vi "Setup subWorker - FPGA Read.vi"(8 "error in":errorcluster, 11 "cRIO NI 9205 Demo in":refnum<class "cRIO NI 9205 Demo.lvclass">) -> (0 "error out":errorcluster, 3 "cRIO NI 9205 Demo out":refnum<class "cRIO NI 9205 Demo.lvclass">)   [LabVIEW 2017, in "cRIO NI 9205 Demo.lvclass"]
doc: "This VI sets up the framework parameters of a statically-linked subWorker."
uses:
  cRIO NI 9205 Demo.lvclass
  cRIO NI 9205 Demo.lvclass/cRIO NI 9205 Demo.ctl
  FPGA Read/FPGA Read.lvclass
  C:/Program Files (x86)/National Instruments/LabVIEW 2017/vi.lib/addons/_Workers/Library/Classes/Worker/Worker.lvclass
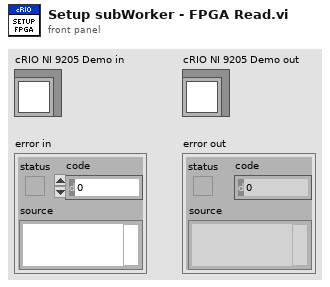
[diagram p1: front panel]
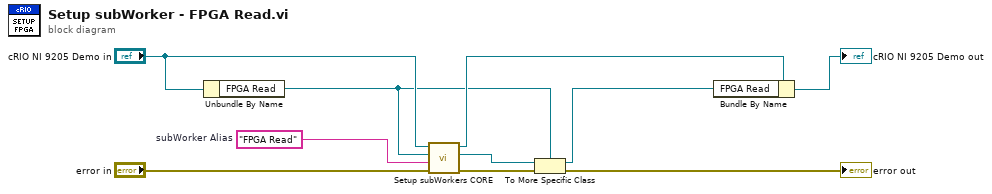
[diagram p0: block diagram]
diagram:
  w6 = "FPGA Read"  # subWorker Alias
  n1 = Unbundle By Name("cRIO NI 9205 Demo in") -> ("FPGA Read"=w3:refnum<class "FPGA Read.lvclass">)
  n2 = call-dynamic "Setup subWorkers CORE.vi"("error in"="error in", "subWorker Alias"=w6, "subWorker"=w3, "Worker"="cRIO NI 9205 Demo in") -> ("error out"=w5:errorcluster, "subWorker out"=w1:refnum<class "Worker.lvclass">, "Worker out"=w8:refnum<class "cRIO NI 9205 Demo.lvclass">)  [unwired: 5 in]
  n3 = To More Specific Class(target class=w3, reference=w1, error in=w5) -> (specific class reference=w2:refnum<class "FPGA Read.lvclass">, error out=→"error out":errorcluster)
  n4 = Bundle By Name(cluster=w8, "FPGA Read"=w2) -> (→"cRIO NI 9205 Demo out":refnum<class "cRIO NI 9205 Demo.lvclass">)
